vi "Digital Write 1 Chan.vi"(8 "Error In":errorcluster, 9 "Output Value":bool, 10 "DO Channel":u8, 11 "LINX Resource":T1) -> (0 "Error Out":errorcluster, 3 "LINX Resource":T1)   [LabVIEW 2020, in "LMH-LINX.lvlib"]
doc: "Write a value to the specified digital output channel."
uses:
  LMH-LINX.lvlib
  Private/Type Defs/Platform.ctl
  Private/Type Defs/Interface.ctl
  Private/Type Defs/LINX Ref.ctl
  Private/Device/Type Defs/Channels.ctl
  Private/Device/Type Defs/TCP Config.ctl
  Private/Device/Device.lvlib
  Private/Device/Type Defs/LINX Device Config.ctl
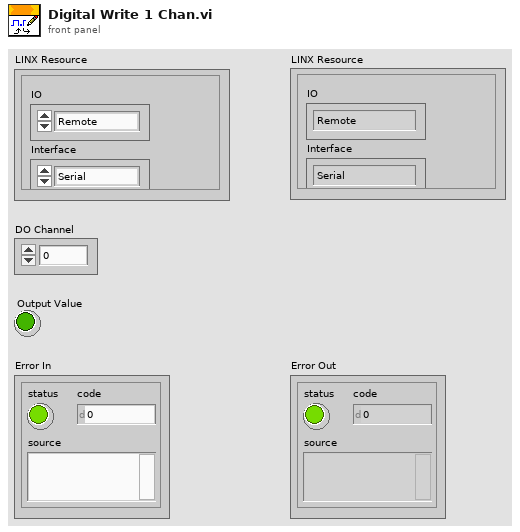
[diagram p1: front panel]
types:
  T1 = typedef "LMH-LINX.lvlib/LINX Ref.ctl" = cluster{"IO":T2, "Interface":T3, "LINX Device Config":T4}
  T2 = typedef "LMH-LINX.lvlib/Platform.ctl" = enum16{"Remote", "Local"}
  T3 = typedef "LMH-LINX.lvlib/Interface.ctl" = enum16{"Serial", "TCP"}
  T4 = typedef "Device.lvlib/LINX Device Config.ctl" = cluster{"Interface":T3, "COM Port":refnum<visa-resource-name>, "TCP Configuration":T5, "Device Family":u8, "Device ID":u8, "Device Name":string, "TCP Ref":refnum<k5>, "Channels":T6}
  T5 = typedef "Device.lvlib/TCP Config.ctl" = cluster{"IP Address":string, "Port":u16}
  T6 = typedef "LMH-LINX.lvlib/Channels.ctl" = cluster{"DI":u8[], "DO":u8[], "AI":u8[], "AO":u8[], "PWM":u8[], "QE":u8[], "UART":u8[], "I2C 2":u8[], "SPI":u8[], "CAN":u8[], "Servo":u8[], "AI Ref (V)":dbl, "AI Resolution (Bits)":u8, "AO Ref (V)":dbl, "AO Resolution (Bits)":u8}
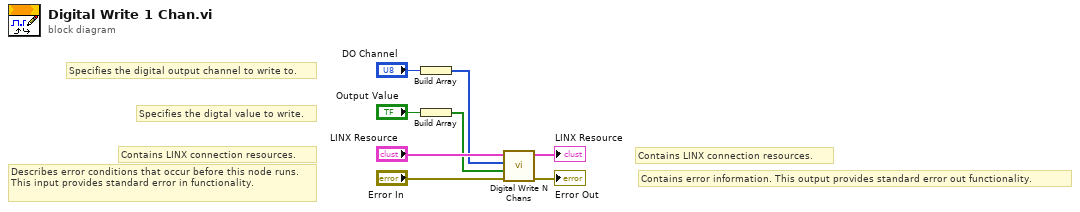
[diagram p0: block diagram]
diagram:
  # "Specifies the digtal value to write."
  # "Specifies the digital output channel to write to."
  # "Contains LINX connection resources."
  # "Contains error information. This output provides standard error out functionality."
  # "Contains LINX connection resources."
  # "Describes error conditions that occur before this node runs. This input provides standard error in functionality."
  n1 = Build Array("DO Channel") -> (w1:u8[])
  n2 = Build Array("Output Value") -> (w2:bool[])
  n3 = call "Digital Write N Chans.vi"("Error In"="Error In", "Values"=w2, "DO Channels"=w1, "LINX Resource"="LINX Resource") -> ("Error Out"=→"Error Out":errorcluster, "LINX Resource"=→"LINX Resource":T1)  [unwired: 6 in]
